vi "Write Nickname.vi"(8 "error in (no error)":errorcluster, 10 "Nickname":string, 11 "Kareem Abdul-Jabbar in":refnum<class "Kareem Abdul-Jabbar.lvclass">) -> (0 "error out":errorcluster, 3 "Kareem Abdul-Jabbar out":refnum<class "Kareem Abdul-Jabbar.lvclass">)   [LabVIEW 2019, in "Kareem Abdul-Jabbar.lvclass"]
uses:
  Kareem Abdul-Jabbar.lvclass
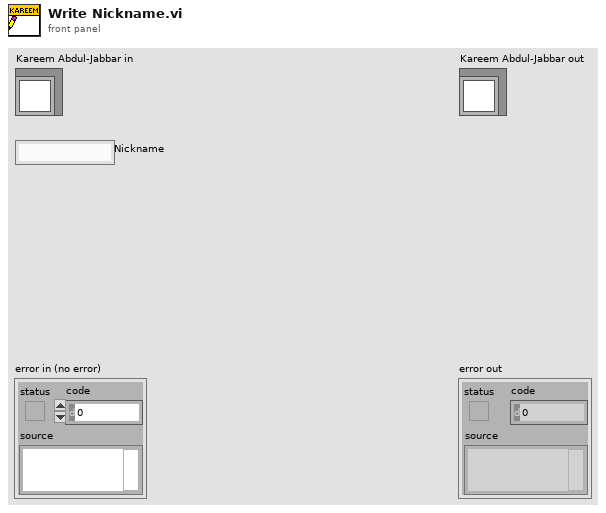
[diagram p1: front panel]
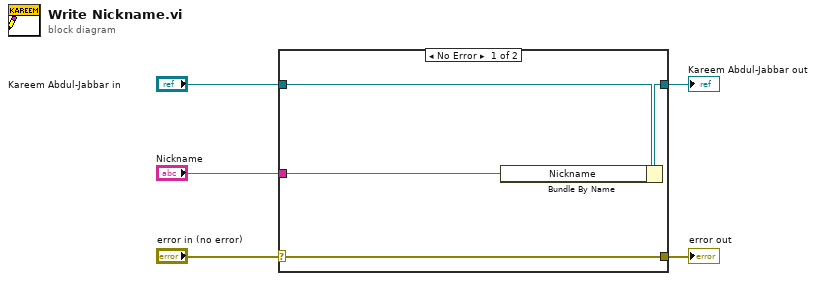
[diagram p0: block diagram]
diagram:
  n1 = case shown="No Error" "error in (no error)" {
    selector: "error in (no error)" -> [w9 w10]
    tunnel: [w9 w10] -> w4
    tunnel: [w7 w11] -> w2
    tunnel: "Kareem Abdul-Jabbar in" -> [w8 w11]
    tunnel: "Nickname" -> [w6 _]
    frame No Error {
      n2 = Bundle By Name(cluster=w8, "Nickname"=w6) -> (w7:refnum<class "Kareem Abdul-Jabbar.lvclass">)
    }
    frame Error {
    }
  }
  "error out" <- w4
  "Kareem Abdul-Jabbar out" <- w2
